vi "Get ParameterName.vi"(11 "Object Type in":refnum<class "Object Type Base.lvclass">) -> (1 "Defined?":bool, 2 "ParameterName":string, 3 "Object Type out":refnum<class "Object Type Base.lvclass">)   [LabVIEW 2024, in "Electronic Datasheet.lvlib" / "Object Type Base.lvclass"]
uses:
  Object Type Base.lvclass
  Object Type Base.lvclass/Object Type Base.ctl
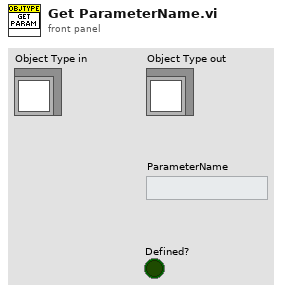
[diagram p1: front panel]
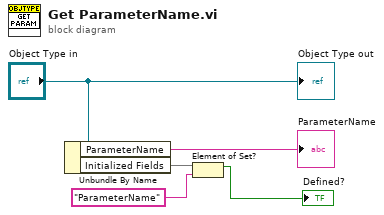
[diagram p0: block diagram]
diagram:
  n1 = Unbundle By Name("Object Type in") -> ("ParameterName"=→"ParameterName":string, "Initialized Fields"=w2:set{string})
  n2 = Element of Set?(10:"ParameterName" ("element"), 11:w2) -> (3:→"Defined?":bool)
  "Object Type out" <- "Object Type in"
